vi "Arduino_Main.vi"   [LabVIEW 2014]
uses:
  <vilib>/Aledyne-TSXperts/Arduino Compatible Compiler for LabVIEW/Code Generator/Arduino APIs/Serial/Serial Settings.ctl
  <vilib>/Aledyne-TSXperts/Arduino Compatible Compiler for LabVIEW/Code Generator/Arduino APIs/I2C/I2C Mode.ctl
  <vilib>/Aledyne-TSXperts/Arduino Compatible Compiler for LabVIEW/Code Generator/Arduino APIs/I2C/I2C Write Array.vi
  <vilib>/Aledyne-TSXperts/Arduino Compatible Compiler for LabVIEW/Arduino Compatible Compiler for LabVIEW.lvlib
types:
  T1 = enum16{"Begin and End", "Begin and Queue", "Queue and End"}
  T2 = typedef "Arduino Compatible Compiler for LabVIEW.lvlib/I2C Mode.ctl" = enum16{"Master", "Slave"}
  T3 = typedef "Arduino Compatible Compiler for LabVIEW.lvlib/Serial Settings.ctl" = u16
  T4 = cluster{"ADS1015-Channel Selector":enum8{"DIFF-AI0-AI1", "DIFF-AI0-AI3", "DIFF-AI1-AI3", "DIFF-AI2-AI3", "Single Ended - AI0", "Single Ended - AI1", "Single Ended - AI2", "Single Ended - AI3"}, "ADS1015 -Gain & Scale":enum8{"FS=+/-6.144 V", "FS=+/-4.096 V", "FS=+/-2.048 V", "FS=+/-1.024 V", "FS=+/-0.512 V", "FS=+/-0.256-A V", "FS=+/-0.256-B V", "FS=+/-0.256-C V"}, "ADS1015- Acquire Mode":enum16{"Continuous Conversion Mode", "Single Shot Mode"}, "ADS1015 Sample Rate":enum8{"128 SPS", "250 SPS", "490 SPS", "920 SPS", "1600 SPS", "2400 SPS", "3300 SPS", "3300 SPS A"}}
  T5 = enum8{"DIFF-AI0-AI1", "DIFF-AI0-AI3", "DIFF-AI1-AI3", "DIFF-AI2-AI3", "Single Ended - AI0", "Single Ended - AI1", "Single Ended - AI2", "Single Ended - AI3"}
  T6 = enum8{"FS=+/-6.144 V", "FS=+/-4.096 V", "FS=+/-2.048 V", "FS=+/-1.024 V", "FS=+/-0.512 V", "FS=+/-0.256-A V", "FS=+/-0.256-B V", "FS=+/-0.256-C V"}
  T7 = enum16{"Continuous Conversion Mode", "Single Shot Mode"}
  T8 = enum8{"128 SPS", "250 SPS", "490 SPS", "920 SPS", "1600 SPS", "2400 SPS", "3300 SPS", "3300 SPS A"}
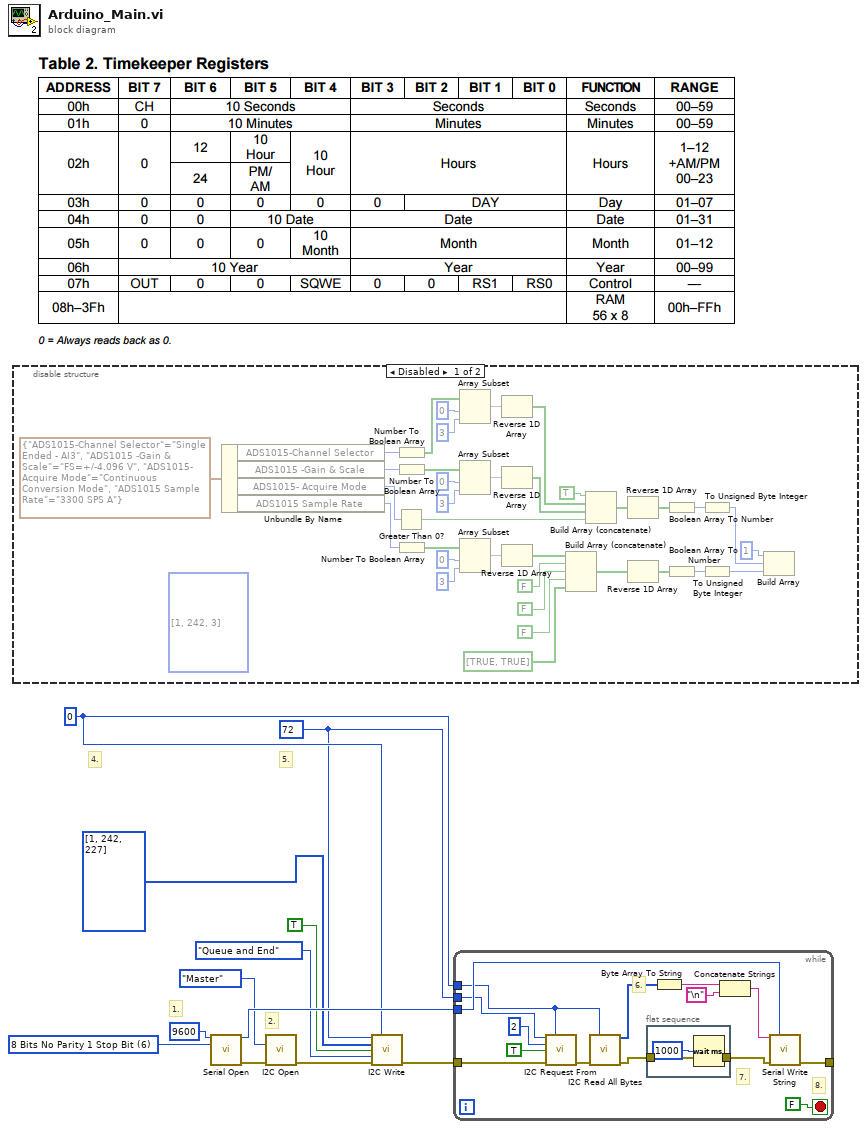
[diagram p0: block diagram]
diagram:
  w7 = u8 0 ("Interface")
  w6 = u8 72 ("Slave Address")
  w10 = T3 6 items=["5 Bits No Parity 1 Stop Bit"=0, "6 Bits No Parity 1 Stop Bit"=2, "7 Bits No Parity 1 Stop Bit"=4, "8 Bits No Parity 1 Stop Bit"=6, "5 Bits No Parity 2 Stop Bits"=8, "6 Bits No Parity 2 Stop Bits"=10, "7 Bits No Parity 2 Stop Bits"=12, "8 Bits No Parity 2 Stop Bits"=14, "5 Bits Even Parity 1 Stop Bits"=32, "6 Bits Even Parity 1 Stop Bits"=34, "7 Bits Even Parity 1 Stop Bits"=36, "8 Bits Even Parity 1 Stop Bits"=38, "5 Bits Even Parity 2 Stop Bits"=40, "6 Bits Even Parity 2 Stop Bits"=42, "7 Bits Even Parity 2 Stop Bits"=44, "8 Bits Even Parity 2 Stop Bits"=46, "5 Bits Odd Parity 1 Stop Bits"=48, "6 Bits Odd Parity 1 Stop Bits"=50, "7 Bits Odd Parity 1 Stop Bits"=52, "8 Bits Odd Parity 1 Stop Bits"=54, "5 Bits Odd Parity 2 Stop Bits"=56, "6 Bits Odd Parity 2 Stop Bits"=58, "7 Bits Odd Parity 2 Stop Bits"=60, "8 Bits Odd Parity 2 Stop Bits"=62] ("Serial Settings")
  # "5."
  # "4."
  # "2."
  # "1."
  n1 = disable-structure shown="Disabled" {
    frame Disabled {
      (unwired) u8[] [1, 242, 3] ("appended array")
      n2 = Unbundle By Name(T4 {"ADS1015-Channel Selector"=enum."Single Ended - AI3", "ADS1015 -Gain & Scale"=enum."FS=+/-4.096 V", "ADS1015- Acquire Mode"=enum."Continuous Conversion Mode", "ADS1015 Sample Rate"=enum."3300 SPS A"} ("ADS1015 Reg Config")) -> ("ADS1015-Channel Selector"=w16:T5, "ADS1015 -Gain & Scale"=w15:T6, "ADS1015- Acquire Mode"=w14:T7, "ADS1015 Sample Rate"=w13:T8)
      n3 = Greater Than 0?(x=w14) -> (x > 0?=w21:bool)
      n4 = Number To Boolean Array(number=w16) -> (Boolean array=w32:bool[])
      n5 = Number To Boolean Array(number=w15) -> (Boolean array=w24:bool[])
      n6 = Number To Boolean Array(number=w13) -> (Boolean array=w47:bool[])
      n7 = Array Subset(array=w32, index=0, length=3) -> (w29:bool[])
      n8 = Array Subset(array=w24, index=0, length=3) -> (w23:bool[])
      n9 = Array Subset(array=w47, index=0, length=3) -> (w44:bool[])
      n10 = Reverse 1D Array(array=w29) -> (reversed array=w27:bool[])
      n11 = Reverse 1D Array(array=w23) -> (reversed array=w22:bool[])
      n12 = Reverse 1D Array(array=w44) -> (reversed array=w43:bool[])
      n13 = Build Array (concatenate)(w43, FALSE, FALSE, FALSE, bool[] [TRUE, TRUE] ("array")) -> (w38:bool[])
      n14 = Build Array (concatenate)(TRUE, w27, w22, w21) -> (w20:bool[])
      n15 = Reverse 1D Array(array=w20) -> (reversed array=w19:bool[])
      n16 = Reverse 1D Array(array=w38) -> (reversed array=w37:bool[])
      n17 = Boolean Array To Number(Boolean array=w19) -> (number=w18:u32)
      n18 = Boolean Array To Number(Boolean array=w37) -> (number=w36:u32)
      n19 = To Unsigned Byte Integer(number=w18) -> (unsigned 8bit integer=w35:u8)
      n20 = To Unsigned Byte Integer(number=w36) -> (unsigned 8bit integer=w33:u8)
      n21 = Build Array(u8 1 ("element"), w35, w33) -> ()  [unwired: 1 out]
    }
    frame Enabled {
    }
  }
  n22 = call <vilib>:"Serial Open.vi"("Speed"=u32 9600, "Serial Settings"=w10) -> ("Instance"=w11:u8, "error out"=w8:errorcluster)  [unwired: 12 in]
  n23 = call <vilib>:"I2C Open.vi"("Mode"=I2C_Mode."Master", "error in (no error)"=w8) -> ("error out"=w3:errorcluster)  [unwired: 12 in, 1 out]
  n24 = call-poly <vilib>:"I2C Write.vi"("Slave Address"=w6, "Interface"=w7, "Data"=u8[] [1, 242, 227] ("appended array"), "Send Stop"=TRUE, "Write Mode"=T1."Queue and End" ("Transmission Type"), "error in (no error)"=w3) -> ("error out"=w5:errorcluster)  [unwired: 8 in, 1 out]
  n25 = while {
    tunnel: [w60] -> _
    tunnel: w11 -> [w61]
    tunnel: w5 -> [w53]
    tunnel: w7 -> [w51]
    tunnel: w6 -> [w54]
    stop <- FALSE stop-if-true
    # "6."
    # "8."
    # "7."
    n26 = call <vilib>:"I2C Request From.vi"("Slave Address"=w54, "Interface"=w51, "Number of Bytes"=u32 2, "Send Stop"=TRUE, "error in (no error)"=w53) -> ("error out"=w50:errorcluster)  [unwired: 10 in]
    n27 = call <vilib>:"I2C Read All Bytes.vi"("Interface"=w51, "error in (no error)"=w50) -> ("Data"=w57:u8[], "error out"=w49:errorcluster)  [unwired: 12 in]
    n28 = flat-sequence {
      tunnel: w49 -> [w64]
      tunnel: [w64] -> w48
      frame #0 {
        n29 = Wait (ms)(milliseconds to wait=u32 1000) -> ()  [unwired: 1 out]
      }
    }
    n30 = Byte Array To String(unsigned byte array=w57) -> (string=w56:string)
    n31 = Concatenate Strings(w56, "\n") -> (w59:string)
    n32 = call <vilib>:"Serial Write String.vi"("String"=w59, "Instance"=w61, "error in (no error)"=w48) -> ("error out"=w60:errorcluster)  [unwired: 12 in]
  }
